vi "AR-Interlock-graph.vi"(11 "Intlk Data Array":T1[](array[typedef]) {"Time Delta (mS)" format="%.3f"}) -> (3 "XY Graph - Dark":cluster{dbl[], i16[]}(graph))   [LabVIEW 2021]
uses:
  Controls/AR-Interlock-Data.ctl
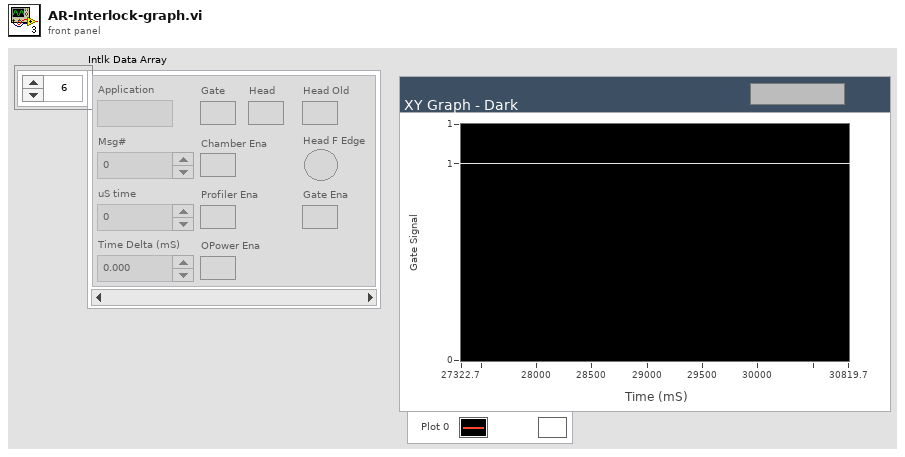
[diagram p1: front panel]
types:
  T1 = typedef "AR-Interlock-Data.ctl" = cluster{"Application":string, "Msg#":i32, "uS time":u32, "Gate":bool, "Head":bool, "Head Old":bool, "Chamber Ena":bool, "Profiler Ena":bool, "OPower Ena":bool, "Gate Ena":bool, "Time Delta (mS)":dbl, "Head F Edge":bool}
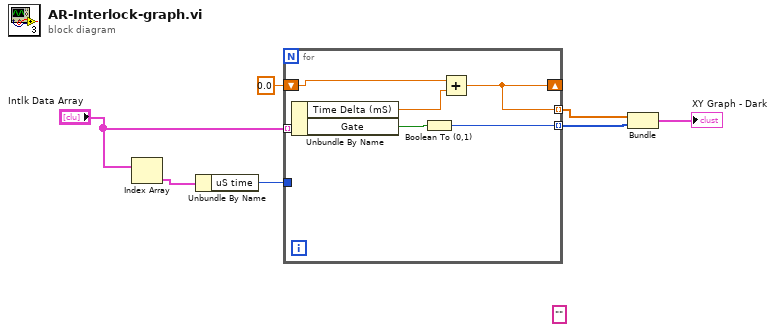
[diagram p0: block diagram]
diagram:
  (unwired) "" ("String")
  n1 = Index Array(array="Intlk Data Array") -> (element=w3:T1)  [unwired: 1 in]
  n2 = Unbundle By Name(w3) -> ("uS time"=w2:u32)
  n3 = for {
    tunnel: "Intlk Data Array" -> [w13] mode=indexing
    tunnel: [w11] -> w7 mode=indexing
    tunnel: [w8] -> w6 mode=indexing
    tunnel: w2 -> [_]
    shift-right: [w8] -> _
    shift-left: 0.0 -> [w9]
    n4 = Unbundle By Name(w13) -> ("Time Delta (mS)"=w10:dbl, "Gate"=w12:bool)
    n5 = Boolean To (0,1)(Boolean=w12) -> (0, 1=w11:i16)
    n6 = Add(x=w9, y=w10) -> (x+y=w8:dbl)
  }
  n7 = Bundle(w6, w7) -> (→"XY Graph - Dark":cluster{dbl[], i16[]})  [unwired: 1 in]
